vi "Get SMO Public API (This Level).vi"(8 "error in (no error)":errorcluster, 11 "Instrument.Framework-Template in":refnum<class "Instrument.Framework-Template.lvclass">) -> (0 "error out":errorcluster, 2 "commands":string[](array[string]), 3 "Instrument.Framework-Template out":refnum<class "Instrument.Framework-Template.lvclass">)   [LabVIEW 2019, in "Instrument.Framework-Template.lvclass"]
doc: "Override this VI to return a list of commands supported by your Instrument"
uses:
  Instrument.Framework-Template.lvclass
  Typedefs/Instrument.Framework-Template.Commands--Enum.ctl
  deb8e169-c360-4423-93ab-b532a9693c4a.vi
  <vilib>/Utility/Data Type/Get Numeric Information.vi
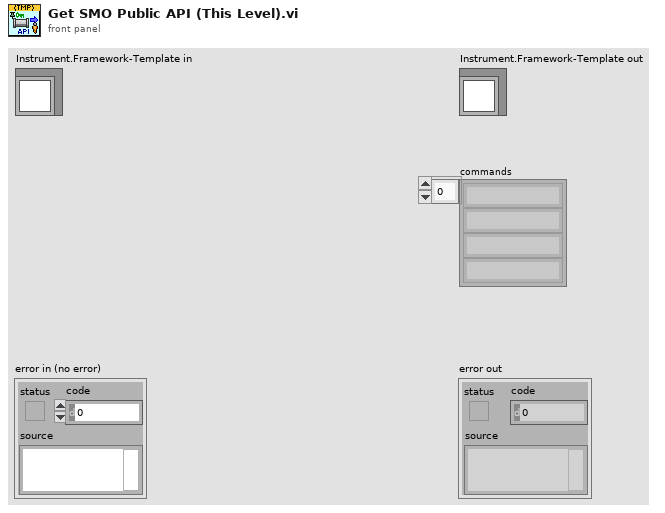
[diagram p1: front panel]
types:
  T1 = typedef "Instrument.Framework-Template.lvclass/Instrument.Framework-Template.Commands--Enum.ctl" = enum16{"doSomething"}
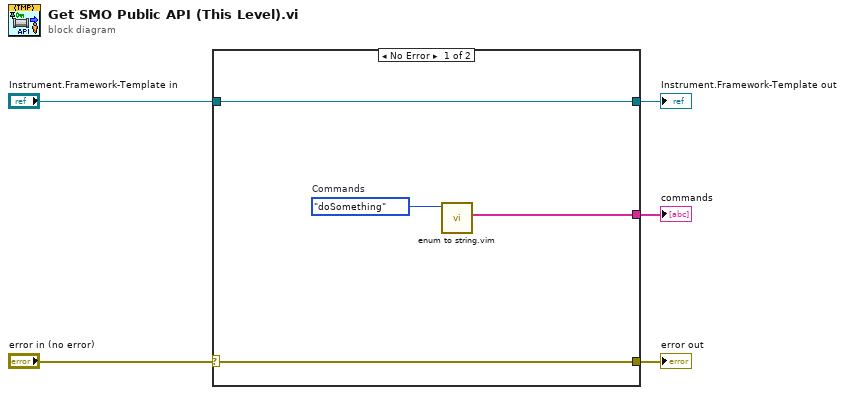
[diagram p0: block diagram]
diagram:
  n1 = case shown="No Error" "error in (no error)" {
    selector: "error in (no error)" -> [w7 w11]
    tunnel: [w8 _] -> w5
    tunnel: [w7 w11] -> w3
    tunnel: [w6 w10] -> w2
    tunnel: "Instrument.Framework-Template in" -> [w6 w10]
    frame No Error {
      w9 = Instrument.Framework-Template.Commands--Enum."doSomething"  # Commands
      n2 = call "enum to string.vim"("enum in"=w9) -> ("strings out"=w8:string[])  [unwired: 9 in, 1 out]
    }
    frame Error {
    }
  }
  "error out" <- w3
  "Instrument.Framework-Template out" <- w2
  "commands" <- w5
